vi "Fetch Receive Transfer Group Inline.vi"(8 "error in (no error)":errorcluster, 10 "Transfer Group in":refnum<class "Transfer Group.lvclass">, 11 "Plugin in":refnum<class "Plugin.lvclass">) -> (0 "error out":errorcluster, 1 "move data?":bool, 2 "Transfer Group out":refnum<class "Transfer Group.lvclass">, 3 "Plugin out":refnum<class "Plugin.lvclass">)   [LabVIEW 2017, in "Data Sharing Framework Core.lvlib" / "Data Sharing Framework Engine.lvlib" / "Plugin.lvclass"]
uses:
  Plugin.lvclass
  Transfer Group/Transfer Group.lvclass
  Transfer Group/Transfer Group.lvclass/Transfer Group.ctl
  Internal/Timing/Engine Timing.lvclass/Engine Timing.ctl
  Internal/Debug/Debug Flags/Debug Flags.lvclass/Debug Flags.ctl
  Internal/Debug/Debug Flags FIFO/Debug Flags FIFO.lvclass/Debug Flags FIFO.ctl
  Transfer Group/Read Return FIFO.vi
  Transfer Group/Get Return FIFO.vi
  Transfer Group/Get Debug Flags.vi
  Internal/Debug/Debug Flags/Get FIFO Flags.vi
  Internal/Debug/Debug Flags FIFO/Get Infinite Timeouts.vi
  Transfer Group/Transfer Group Errors.vi
  Transfer Group/Return Timeout Error.vi
  Internal/Timing/Engine Timing.lvclass
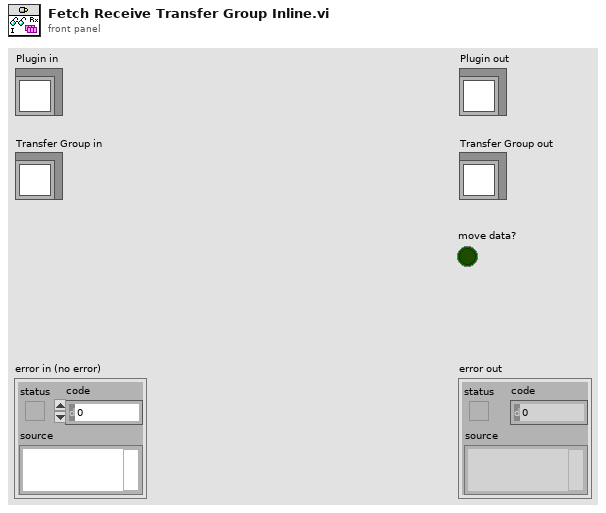
[diagram p1: front panel]
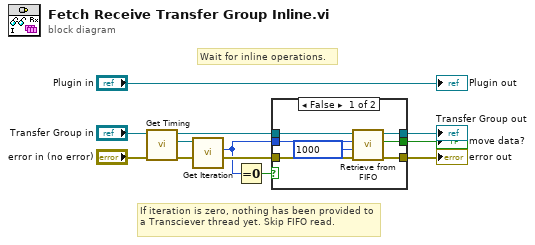
[diagram p0: block diagram]
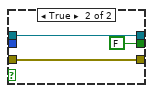
[diagram p2: hidden frame]
diagram:
  # "Wait for inline operations."
  # "If iteration is zero, nothing has been provided to a Transciever thread yet. Skip FIFO read."
  n1 = call "Get Timing.vi"("Transfer Group in"="Transfer Group in") -> ("Timing"=w4:refnum<class "Engine Timing.lvclass">, "Transfer Group out"=w5:refnum<class "Transfer Group.lvclass">)  [unwired: 9 in]
  n2 = call "Get Iteration.vi"("Timing in"=w4) -> ("Iteration"=w3:u64)  [unwired: 9 in, 1 out]
  n3 = Equal To 0?(x=w3) -> (x = 0?=w2:bool)
  n4 = case shown="False" w2 {
    tunnel: "error in (no error)" -> [w17 w19]
    tunnel: [w16 w20] -> w9
    tunnel: [w15 w19] -> w8
    tunnel: w5 -> [w14 w20]
    tunnel: w3 -> [w13 _]
    tunnel: [w12 FALSE ("iteration valid?")] -> w1
    frame False {
      n5 = call "Retrieve from FIFO.vi"("error in (no error)"=w17, "timeout in ms (0)"=1000, "expected iteration"=w13, "Transfer Group in"=w14) -> ("error out"=w15:errorcluster, "iteration valid?"=w12:bool, "Transfer Group out"=w16:refnum<class "Transfer Group.lvclass">)  [unwired: 5 in]
    }
    frame True {
    }
  }
  "error out" <- w8
  "Transfer Group out" <- w9
  "move data?" <- w1
  "Plugin out" <- "Plugin in"
